vi "Extract Array Thresholds.vi"(9 "data":dbl[](array[numeric]), 10 "Lower Threshold (% of Min)":dbl=120.0, 11 "Upper Threshold (% of Max)":dbl=80.0) -> (0 "Lower  Subarray":dbl[](array[numeric]), 1 "Upper Subarray":dbl[](array[numeric]), 2 "Lower Voltage Threshold":dbl, 3 "Upper Voltage Threshold":dbl)   [LabVIEW 2009]
panel:
  out "Waveform Graph":dbl[](graph)
  out "size(s)":i32
  out "max value":dbl
  out "min value":dbl
  out "Lower Delete Length":i32
  out "Upper Delete Length":i32
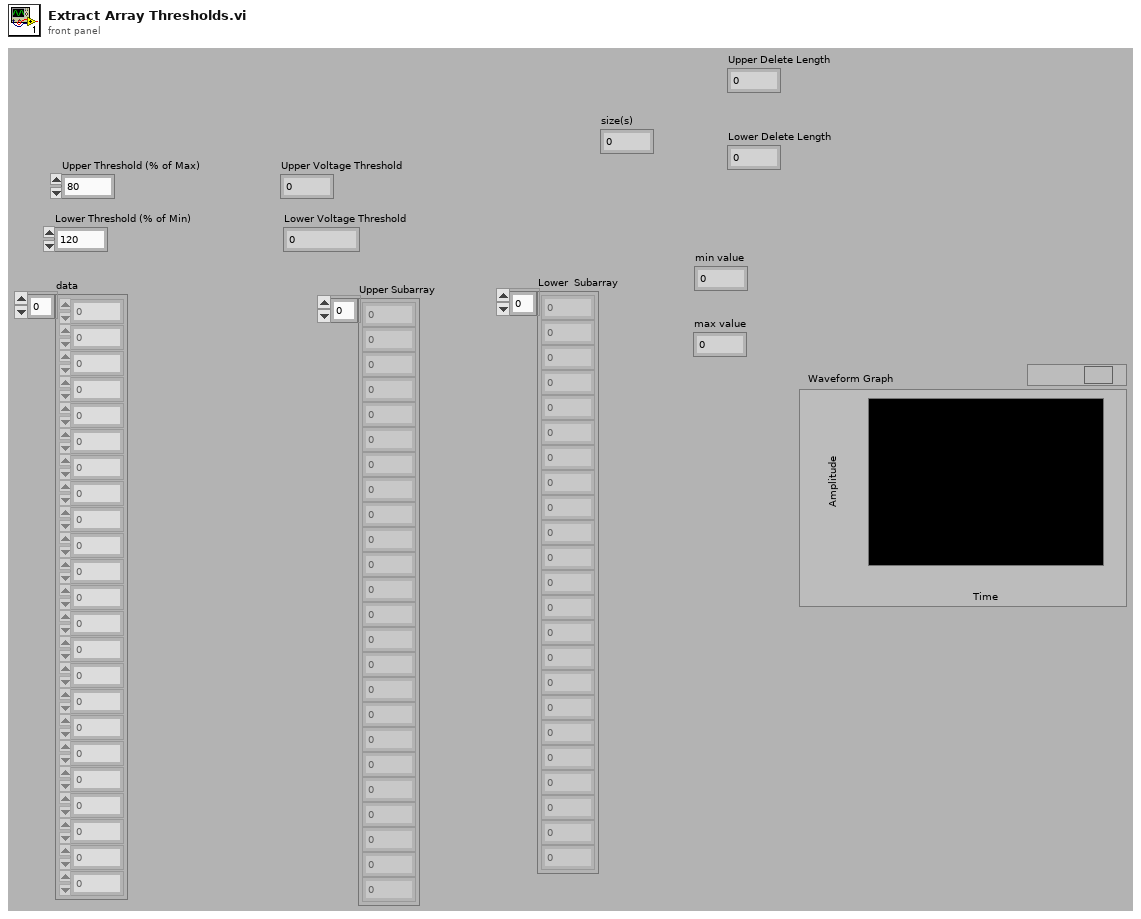
[diagram p1: front panel]
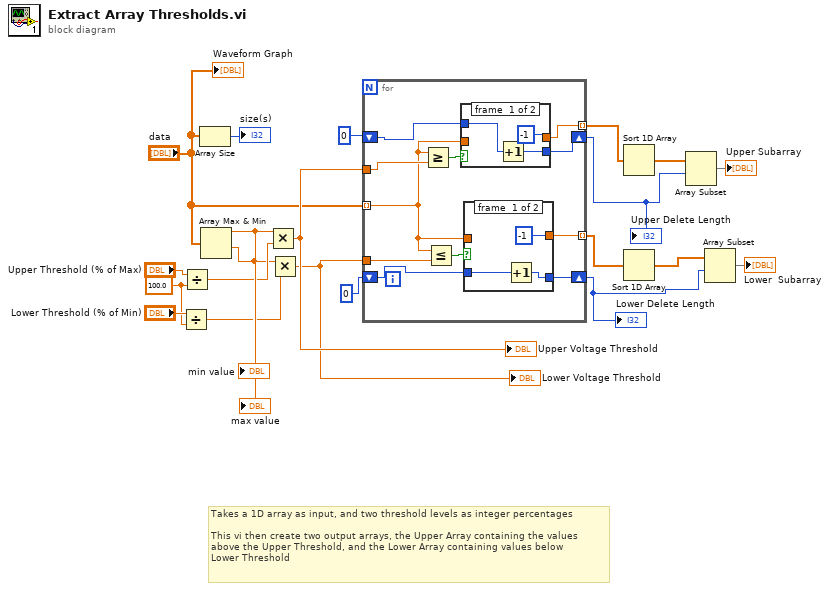
[diagram p0: block diagram]
diagram:
  w17 = 100.0 ("y")
  # "Takes a 1D array as input, and two threshold levels as integer percentages\n\nThis vi then create two output arrays, the Upper Array containing the values\nabove the Upper Threshold, and the Lower Array containing values below \nLower Threshold"
  n1 = Divide(x="Lower Threshold (% of Min)", y=w17) -> (x/y=w15:dbl)
  n2 = Divide(x="Upper Threshold (% of Max)", y=w17) -> (x/y=w19:dbl)
  n3 = Array Size(array="data") -> (size(s)=→"size(s)":i32)
  n4 = Array Max & Min(array="data") -> (max value=w21:dbl, min value=w16:dbl)  [unwired: 2 out]
  "min value" <- w16
  "max value" <- w21
  n5 = Multiply(x=w21, y=w19) -> (x*y=w14:dbl)
  "Upper Voltage Threshold" <- w14
  n6 = Multiply(x=w16, y=w15) -> (x*y=w13:dbl)
  "Lower Voltage Threshold" <- w13
  n7 = for {
    tunnel: "data" -> [w27] mode=indexing
    tunnel: w14 -> [w32]
    tunnel: w13 -> [w28]
    shift-right: [w24] -> w3
    shift-left: 0 -> [w25]
    shift-right: [w22] -> w4
    shift-left: 0 -> [w23]
    tunnel: [w26] -> w9 mode=indexing
    tunnel: [w30] -> w10 mode=indexing
    n8 = Greater Or Equal?(x=w27, y=w32) -> (x >= y?=w31:bool)
    n9 = Less Or Equal?(x=w27, y=w28) -> (x <= y?=w29:bool)
    n10 = case shown="True" w31 {
      tunnel: w27 -> [_ w41]
      tunnel: [-1 w41] -> w30
      tunnel: w23 -> [w40 w42]
      tunnel: [w39 w42] -> w22
      frame #0 {
        n11 = Increment(x=w40) -> (x+1=w39:i32)
      }
      frame #1 {
      }
    }
    n12 = case shown="True" w29 {
      tunnel: [-1 w36] -> w26
      tunnel: w27 -> [_ w36]
      tunnel: w25 -> [w35 w37]
      tunnel: [w34 w37] -> w24
      frame #0 {
        n13 = Increment(x=w35) -> (x+1=w34:i32)
      }
      frame #1 {
      }
    }
  }
  "Upper Delete Length" <- w4
  "Lower Delete Length" <- w3
  n14 = Sort 1D Array(array=w10) -> (sorted array=w8:dbl[])
  n15 = Sort 1D Array(array=w9) -> (sorted array=w5:dbl[])
  n16 = Array Subset(array=w8, index=w4) -> (→"Upper Subarray":dbl[])  [unwired: 1 in]
  n17 = Array Subset(array=w5, index=w3) -> (→"Lower  Subarray":dbl[])  [unwired: 1 in]
  "Waveform Graph" <- "data"
